vi "Resolve Name.vi"(10 "Name in":string, 11 "Channels":T2[](array[typedef])) -> (2 "Name out":string, 3 "Connection":T1 {"Custom Data" format="%.0x"})   [LabVIEW 2021, in "CIFCoreWrapper.lvlib"]
uses:
  CIFCoreWrapper.lvlib
  CIFCoreChannel_client/RPC Messages/cif_channelcore_Channel.ctl
  CIFCoreChannel_client/RPC Messages/cif_channelcore_Direction.ctl
  CIFCoreChannel_client/RPC Messages/cif_channelcore_PATTERN.ctl
  <vilib>/CIF Foundation/CIF Channels Core/ChannelCommon/typedef/New FIFO Instance Response.ctl
  <vilib>/CIF Foundation/CIF Channels Core/ChannelCommon/ChannelCommon.lvlib
  CIFCoreChannel_client/CIFCoreChannel_client.lvlib
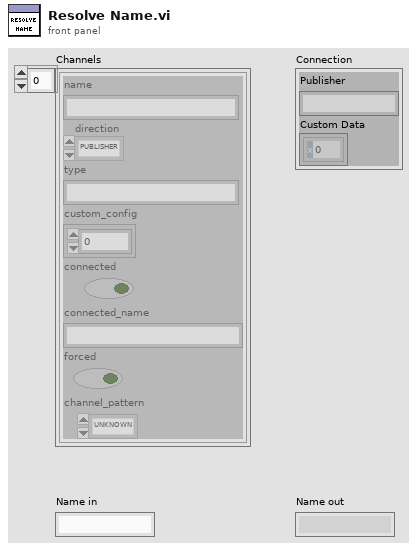
[diagram p1: front panel]
types:
  T1 = typedef "ChannelCommon.lvlib/New FIFO Instance Response.ctl" = cluster{"Publisher":string, "Custom Data":u8[]}
  T2 = typedef "CIFCoreChannel_client.lvlib/cif_channelcore_Channel.ctl" = cluster{"name":string, "direction":T3, "type":string, "custom_config":u8[], "connected":bool, "connected_name":string, "forced":bool, "channel_pattern":T4}
  T3 = typedef "CIFCoreChannel_client.lvlib/cif_channelcore_Direction.ctl" = enum32{"PUBLISHER", "SUBSCRIBER"}
  T4 = typedef "CIFCoreChannel_client.lvlib/cif_channelcore_PATTERN.ctl" = enum32{"UNKNOWN", "TAG", "FIFO", "MULTIFIFO", "BACKPRESSUREFIFO"}
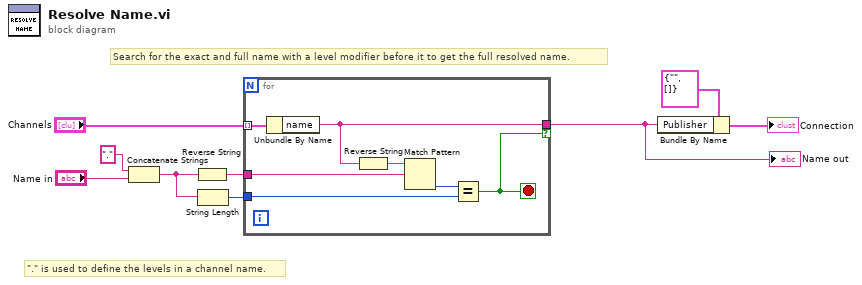
[diagram p0: block diagram]
diagram:
  # "Search for the exact and full name with a level modifier before it to get the full resolved name."
  # "\".\" is used to define the levels in a channel name."
  n1 = Concatenate Strings("." ("string"), "Name in") -> (w6:string)
  n2 = Reverse String(1:w6) -> (0:w8:string)
  n3 = String Length(string=w6) -> (length=w9:i32)
  n4 = for {
    tunnel: "Channels" -> [w16] mode=indexing
    tunnel: [w14] -> w1 if=w12
    tunnel: w9 -> [w11]
    tunnel: w8 -> [w10]
    stop <- w12 stop-if-true
    n5 = Unbundle By Name(w16) -> ("name"=w14:string)
    n6 = Reverse String(1:w14) -> (0:w15:string)
    n7 = Match Pattern(string=w15, regular expression=w10) -> (offset past match=w13:i32)  [unwired: 1 in, 3 out]
    n8 = Equal?(x=w13, y=w11) -> (x = y?=w12:bool)
  }
  "Name out" <- w1
  n9 = Bundle By Name(cluster=T1 {"Publisher"="", "Custom Data"=[]} ("Connection"), "Publisher"=w1) -> (→"Connection":T1)
